vi "image2picture.vi"(8 "error in (no error)":errorcluster, 11 "data_loader in":refnum<class "data_loader.lvclass">) -> (0 "error out":errorcluster, 3 "data_loader out":refnum<class "data_loader.lvclass">)   [LabVIEW 2017, in "data_loader.lvclass"]
uses:
  data_loader.lvclass
  data_loader.lvclass/data_loader.ctl
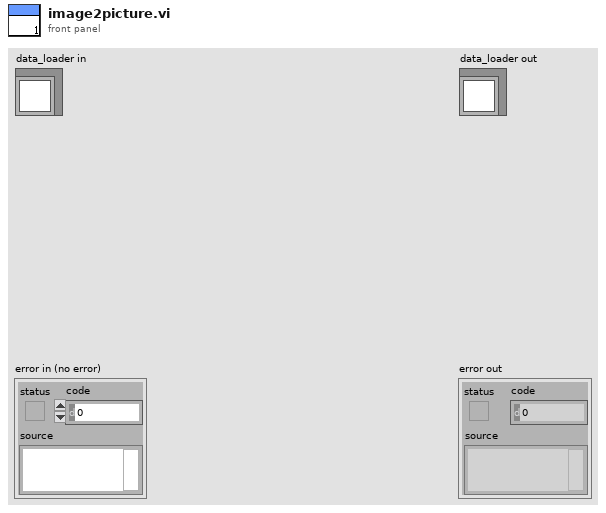
[diagram p1: front panel]
types:
  T1 = typedef "IMAQ Image.ctl" = refnum<image>
  T2 = typedef "imagedata.ctl" = cluster{"image type":i32, "image depth":i32, "image":u8[], "mask":u8[], "colors":u32[], "Rectangle":cluster{"left":i16, "top":i16, "right":i16, "bottom":i16}}
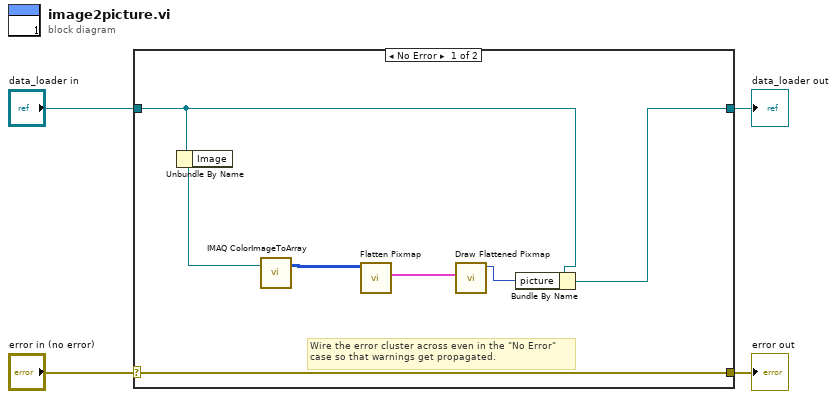
[diagram p0: block diagram]
diagram:
  n1 = case shown="No Error" "error in (no error)" {
    selector: "error in (no error)" -> [w11 w13]
    tunnel: [w11 w13] -> w3
    tunnel: [w5 w12] -> w1
    tunnel: "data_loader in" -> [w6 w12]
    frame No Error {
      # "Wire the error cluster across even in the \"No Error\"\ncase so that warnings get propagated."
      n2 = Unbundle By Name(w6) -> ("Image"=w10:T1)
      n3 = call "IMAQ ColorImageToArray"("Image"=w10) -> ("Image Pixels (U32)"=w9:u32[][])  [unwired: 3 in, 2 out]
      n4 = call <vilib>:"Flatten Pixmap.vi"("24-bit pixmap"=w9) -> ("image data"=w8:T2)  [unwired: 10 in]
      n5 = call <vilib>:"Draw Flattened Pixmap.vi"("image data"=w8) -> ("new picture"=w7:picture)  [unwired: 8 in]
      n6 = Bundle By Name(cluster=w6, "picture"=w7) -> (w5:refnum<class "data_loader.lvclass">)
    }
    frame Error {
    }
  }
  "error out" <- w3
  "data_loader out" <- w1
